vi "uid.get.vi"(8 "error in (no error)":errorcluster, 11 "midi-file-events in":refnum<class "midi-file-event.lvclass">) -> (0 "error out":errorcluster, 2 "uid":string, 3 "midi-file-events out":refnum<class "midi-file-event.lvclass">)   [LabVIEW 2020, in "midi-file-event.lvclass"]
uses:
  midi-file-event.lvclass
  midi-file-event.lvclass/midi-file-event.ctl
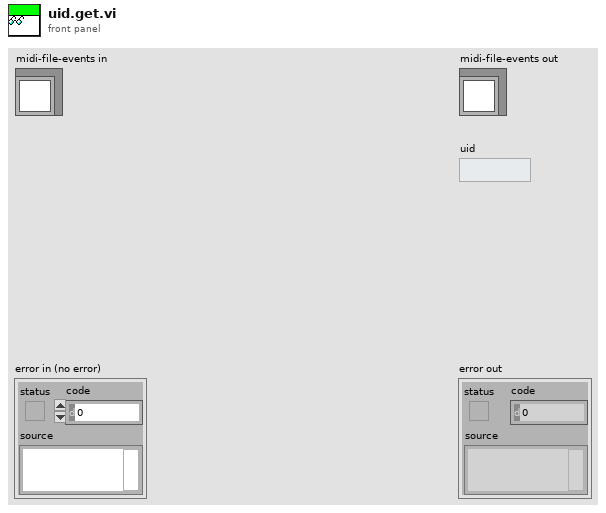
[diagram p1: front panel]
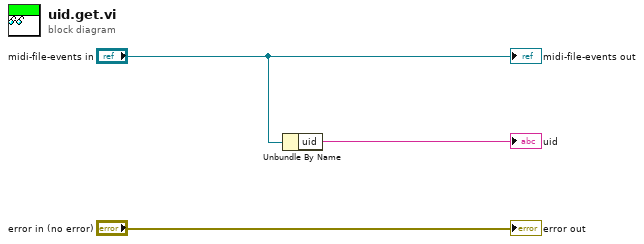
[diagram p0: block diagram]
diagram:
  n1 = Unbundle By Name("midi-file-events in") -> ("uid"=→"uid":string)
  "error out" <- "error in (no error)"
  "midi-file-events out" <- "midi-file-events in"
